vi "Replace timestamp.vi"(10 "Array in (use this time stamp)":waveform(dbl)[](array[waveform]), 11 "Array in":waveform(dbl)[](array[waveform])) -> (3 "Array out":waveform(dbl)[](array[waveform]))   [LabVIEW 2019, in "Instrument.DAQ.lvclass"]
uses:
  Instrument.DAQ.lvclass
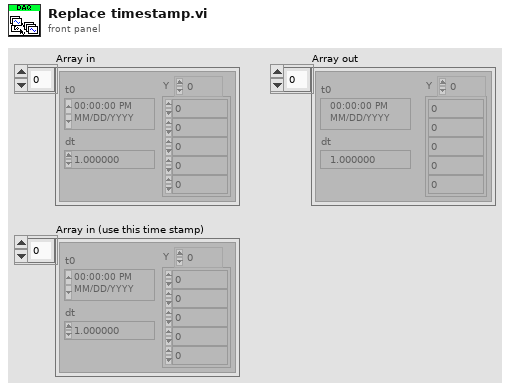
[diagram p1: front panel]
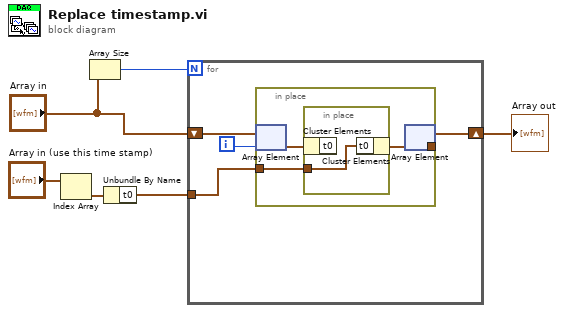
[diagram p0: block diagram]
diagram:
  n1 = Index Array(array="Array in (use this time stamp)") -> (element=w4:waveform(dbl))  [unwired: 1 in]
  n2 = Array Size(array="Array in") -> (size(s)=w6:i32)
  n3 = Unbundle By Name(w4) -> ("t0"=w2:timestamp)
  n4 = for {
    N: w6 -> [_]
    shift-right: [w8] -> w5
    shift-left: "Array in" -> [w10]
    tunnel: w2 -> [w7]
    i -> [w9]
    n5 = in-place {
      in-place-border: w7 -> [w12]
      in-place-border: [w11] -> _
      n6 = in-place-array #1(w10, w9) -> (w13:waveform(dbl))
      n7 = in-place {
        in-place-border: w12 -> [w14]
        n8 = in-place-cluster #2(w13) -> ()  [unwired: 1 out]
        n9 = in-place-cluster #2("t0"=w14) -> (w11:waveform(dbl))
      }
      n10 = in-place-array #1(w11) -> (w8:waveform(dbl)[])  [unwired: 1 out]
    }
  }
  "Array out" <- w5
